vi "ForceAnnotationAuto.vi"(4 "EnReturnForce":bool, 5 "EnFullAngle":bool, 6 "SpectConfig":T4, 7 "FirstTouch":T3={"FirstPeakforce"=2.0, "F_LengthView"=20, "A_LengthView "=20} {"FirstPeakforce" format="%#_13g"}, 8 "ShowName":cluster{"ShowArrow":bool, "Alias":bool}, 9 "Test Name":string(combo)="WDW", 10 "Graph Up":refnum<vi>, 11 "Graph Down":refnum<vi>) -> (0 "MaxForceUp":T2, 1 "ResultUp":T1, 2 "ResultDown":T1, 3 "MaxForceDown":T2)   [LabVIEW 2017]
uses:
  <vilib>/Utility/miscctls.llb/LVAnnotationListTypeDef.ctl
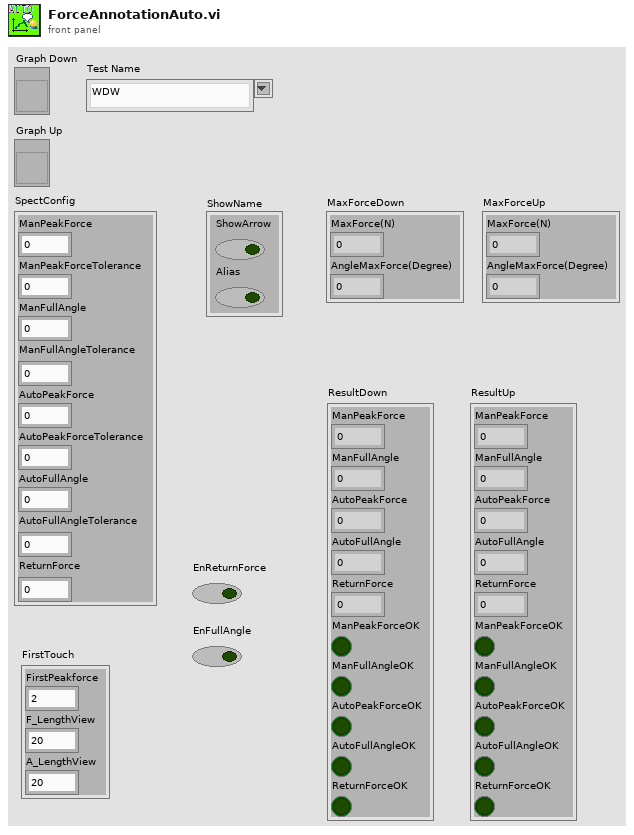
[diagram p1: front panel]
types:
  T1 = cluster{"ManPeakForce":dbl, "ManFullAngle":dbl, "AutoPeakForce":dbl, "AutoFullAngle":dbl, "ReturnForce":dbl, "ManPeakForceOK":bool, "ManFullAngleOK":bool, "AutoPeakForceOK":bool, "AutoFullAngleOK":bool, "ReturnForceOK":bool}
  T2 = cluster{"MaxForce(N)":dbl, "AngleMaxForce(Degree)":dbl}
  T3 = cluster{"FirstPeakforce":dbl, "F_LengthView":i32, "A_LengthView ":i32}
  T4 = cluster{"ManPeakForce":dbl, "ManPeakForceTolerance":dbl, "ManFullAngle":dbl, "ManFullAngleTolerance":dbl, "AutoPeakForce":dbl, "AutoPeakForceTolerance":dbl, "AutoFullAngle":dbl, "AutoFullAngleTolerance":dbl, "ReturnForce":dbl}
  T5 = cluster{"FirstForce":dbl, "LengthView":i32, "Name":string}
  T6 = typedef "LVAnnotationListTypeDef.ctl" = cluster{"Name":string, "Color":u32, "Style":u8, "Point Style":u8, "Name Visible":bool, "Allow Drag":bool, "Annotation Mode":u32, "Plot":i32, "Index":i32, "Position":cluster{"X":dbl, "Y":dbl}, "X Scale":u32, "Y Scale":u32, "Show Arrow":bool, "Lock Name":bool, "Plot Area":i32, "Label Offset":cluster{"X":dbl, "Y":dbl}}[]
  T7 = cluster{"Annotation List[0]":cluster{"Name":string, "Color":u32, "Style":u8, "Point Style":u8, "Name Visible":bool, "Allow Drag":bool, "Annotation Mode":u32, "Plot":i32, "Index":i32, "Position":cluster{"X":dbl, "Y":dbl}, "X Scale":u32, "Y Scale":u32, "Show Arrow":bool, "Lock Name":bool, "Plot Area":i32, "Label Offset":cluster{"X":dbl, "Y":dbl}}, "Annotation List[1]":cluster{"Name":string, "Color":u32, "Style":u8, "Point Style":u8, "Name Visible":bool, "Allow Drag":bool, "Annotation Mode":u32, "Plot":i32, "Index":i32, "Position":cluster{"X":dbl, "Y":dbl}, "X Scale":u32, "Y Scale":u32, "Show Arrow":bool, "Lock Name":bool, "Plot Area":i32, "Label Offset":cluster{"X":dbl, "Y":dbl}}, "Annotation List[2]":cluster{"Name":string, "Color":u32, "Style":u8, "Point Style":u8, "Name Visible":bool, "Allow Drag":bool, "Annotation Mode":u32, "Plot":i32, "Index":i32, "Position":cluster{"X":dbl, "Y":dbl}, "X Scale":u32, "Y Scale":u32, "Show Arrow":bool, "Lock Name":bool, "Plot Area":i32, "Label Offset":cluster{"X":dbl, "Y":dbl}}, "Annotation List[3]":cluster{"Name":string, "Color":u32, "Style":u8, "Point Style":u8, "Name Visible":bool, "Allow Drag":bool, "Annotation Mode":u32, "Plot":i32, "Index":i32, "Position":cluster{"X":dbl, "Y":dbl}, "X Scale":u32, "Y Scale":u32, "Show Arrow":bool, "Lock Name":bool, "Plot Area":i32, "Label Offset":cluster{"X":dbl, "Y":dbl}}, "Annotation List[4]":cluster{"Name":string, "Color":u32, "Style":u8, "Point Style":u8, "Name Visible":bool, "Allow Drag":bool, "Annotation Mode":u32, "Plot":i32, "Index":i32, "Position":cluster{"X":dbl, "Y":dbl}, "X Scale":u32, "Y Scale":u32, "Show Arrow":bool, "Lock Name":bool, "Plot Area":i32, "Label Offset":cluster{"X":dbl, "Y":dbl}}, "Annotation List[5]":cluster{"Name":string, "Color":u32, "Style":u8, "Point Style":u8, "Name Visible":bool, "Allow Drag":bool, "Annotation Mode":u32, "Plot":i32, "Index":i32, "Position":cluster{"X":dbl, "Y":dbl}, "X Scale":u32, "Y Scale":u32, "Show Arrow":bool, "Lock Name":bool, "Plot Area":i32, "Label Offset":cluster{"X":dbl, "Y":dbl}}, "Annotation List[6]":cluster{"Name":string, "Color":u32, "Style":u8, "Point Style":u8, "Name Visible":bool, "Allow Drag":bool, "Annotation Mode":u32, "Plot":i32, "Index":i32, "Position":cluster{"X":dbl, "Y":dbl}, "X Scale":u32, "Y Scale":u32, "Show Arrow":bool, "Lock Name":bool, "Plot Area":i32, "Label Offset":cluster{"X":dbl, "Y":dbl}}, "Annotation List[7]":cluster{"Name":string, "Color":u32, "Style":u8, "Point Style":u8, "Name Visible":bool, "Allow Drag":bool, "Annotation Mode":u32, "Plot":i32, "Index":i32, "Position":cluster{"X":dbl, "Y":dbl}, "X Scale":u32, "Y Scale":u32, "Show Arrow":bool, "Lock Name":bool, "Plot Area":i32, "Label Offset":cluster{"X":dbl, "Y":dbl}}, "Annotation List[8]":cluster{"Name":string, "Color":u32, "Style":u8, "Point Style":u8, "Name Visible":bool, "Allow Drag":bool, "Annotation Mode":u32, "Plot":i32, "Index":i32, "Position":cluster{"X":dbl, "Y":dbl}, "X Scale":u32, "Y Scale":u32, "Show Arrow":bool, "Lock Name":bool, "Plot Area":i32, "Label Offset":cluster{"X":dbl, "Y":dbl}}}
  T8 = cluster{"Name":string, "Color":u32, "Style":u8, "Point Style":u8, "Name Visible":bool, "Allow Drag":bool, "Annotation Mode":u32, "Plot":i32, "Index":i32, "Position":cluster{"X":dbl, "Y":dbl}, "X Scale":u32, "Y Scale":u32, "Show Arrow":bool, "Lock Name":bool, "Plot Area":i32, "Label Offset":cluster{"X":dbl, "Y":dbl}}[]
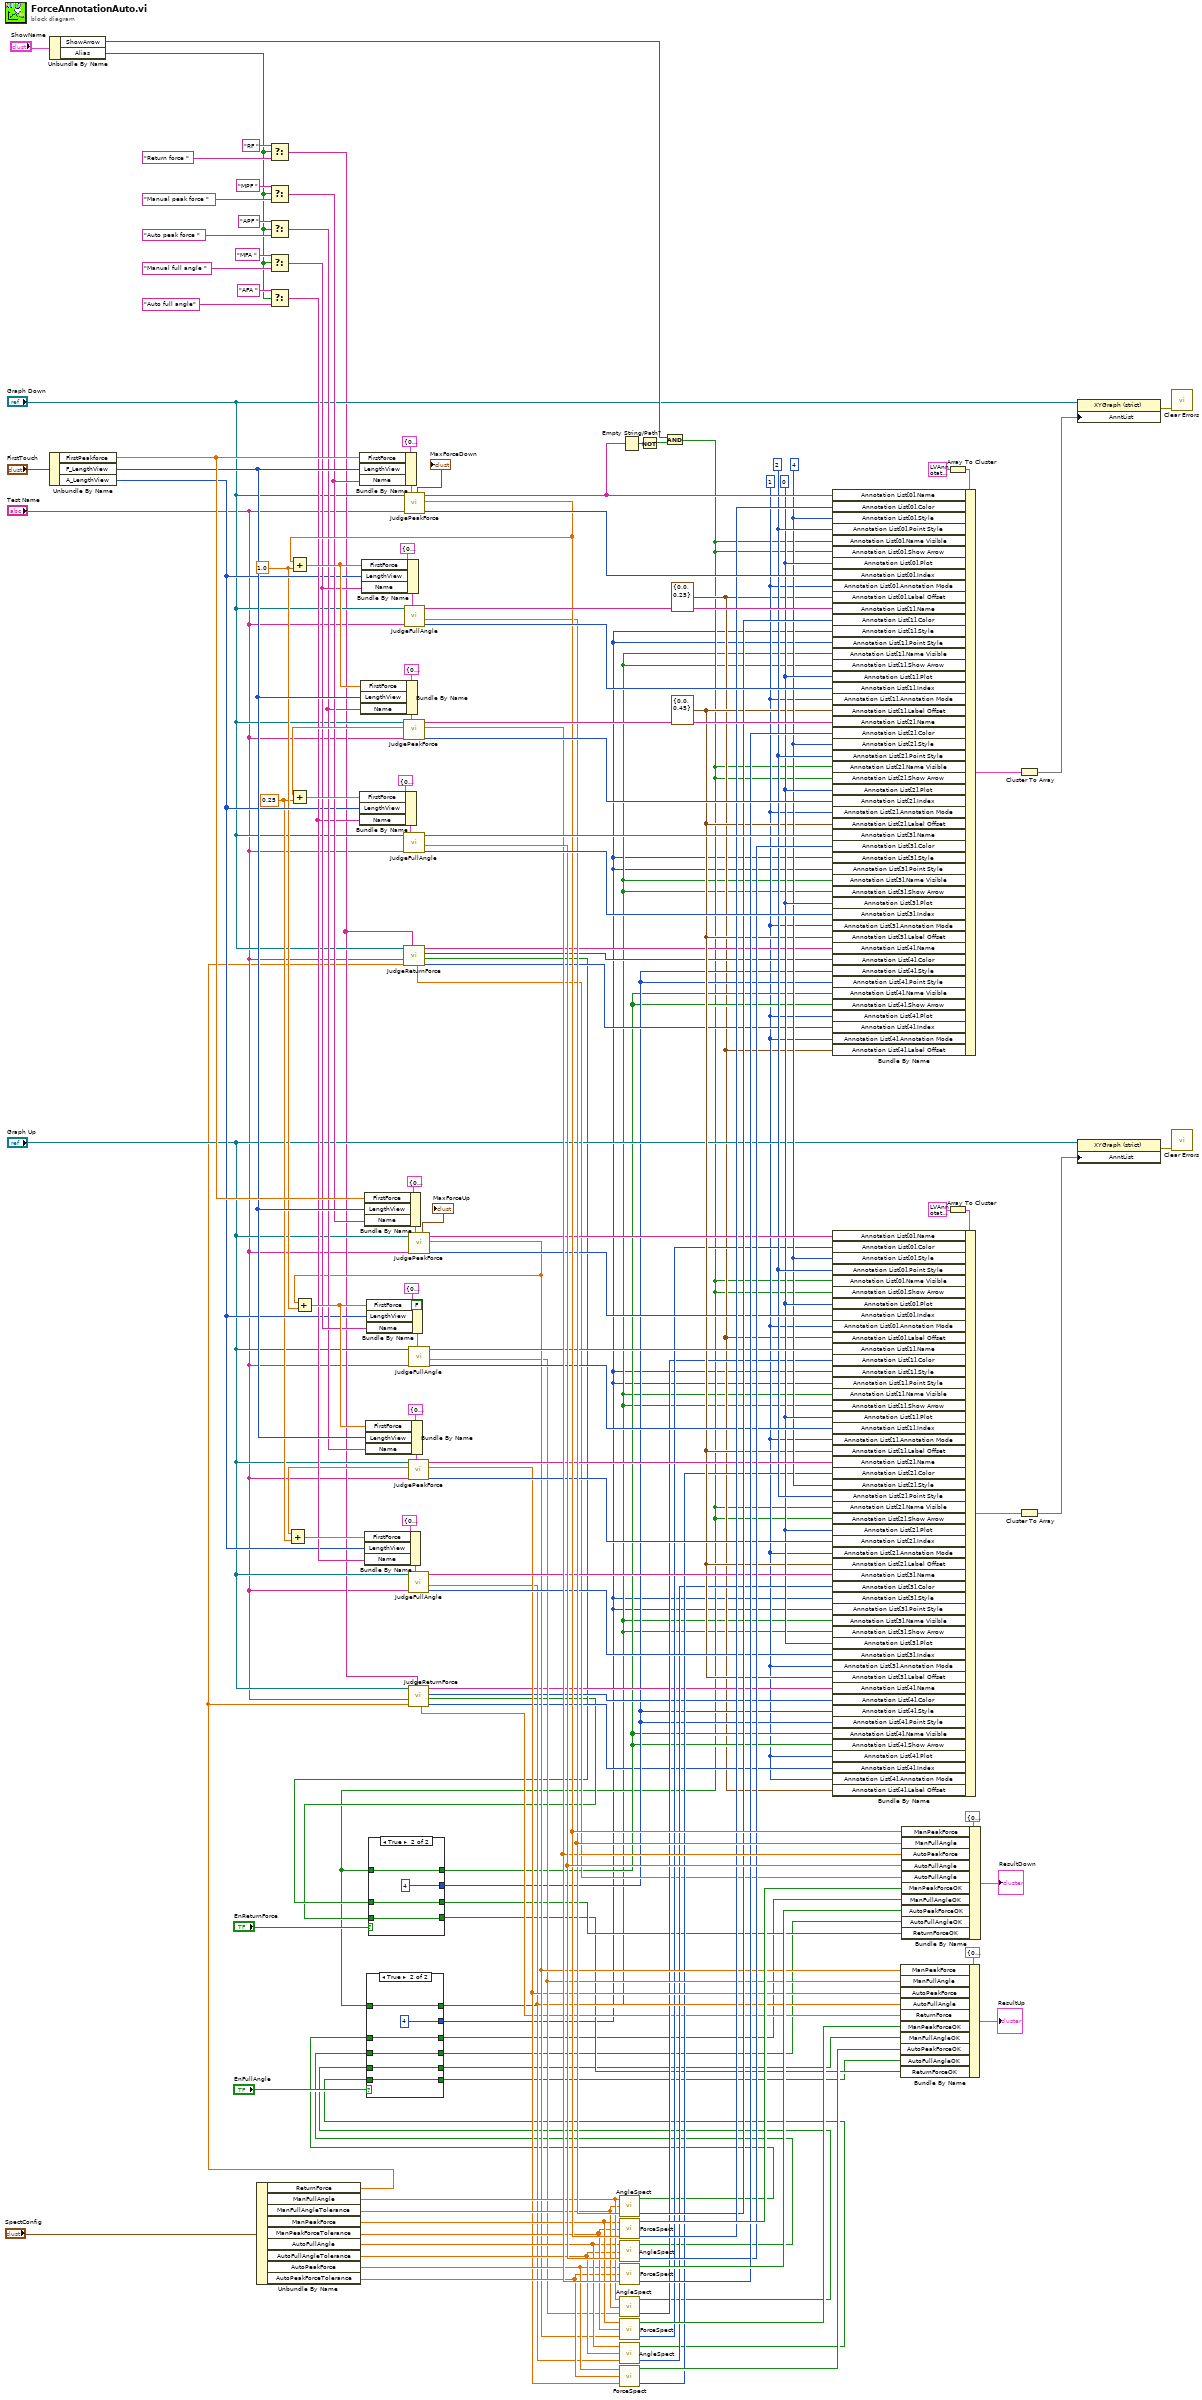
[diagram p0: block diagram]
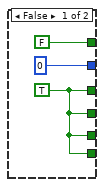
[diagram p2: hidden frame]
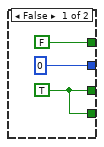
[diagram p3: hidden frame]
diagram:
  (unwired) FALSE ("Auto")
  w71 = 0 ("Annotation List[0].Plot")
  w69 = cluster{"X":dbl, "Y":dbl} {"X"=0.0, "Y"=0.45} ("Annotation List[0].Label Offset")
  w42 = 0.25 ("y")
  w43 = 1.0 ("y")
  w72 = u8 2 ("Annotation List[0].Point Style")
  w17 = cluster{"X":dbl, "Y":dbl} {"X"=0.0, "Y"=0.25} ("Annotation List[0].Label Offset")
  w18 = u32 1 ("Annotation List[0].Annotation Mode")
  w70 = u8 4 ("Annotation List[0].Style")
  n1 = Unbundle By Name("FirstTouch") -> ("FirstPeakforce"=w68:dbl, "F_LengthView"=w67:i32, "A_LengthView"=w62:i32)
  n2 = Unbundle By Name("ShowName") -> ("ShowArrow"=w127:bool, "Alias"=w38:bool)
  n3 = Unbundle By Name("SpectConfig") -> ("ReturnForce"=w25:dbl, "ManFullAngle"=w61:dbl, "ManFullAngleTolerance"=w60:dbl, "ManPeakForce"=w59:dbl, "ManPeakForceTolerance"=w58:dbl, "AutoFullAngle"=w57:dbl, "AutoFullAngleTolerance"=w56:dbl, "AutoPeakForce"=w55:dbl, "AutoPeakForceTolerance"=w54:dbl)
  n4 = Select(t="RF ", s=w38, f="Return force " ("Name")) -> (s? t:f=w27:string)
  n5 = Select(t="MPF ", s=w38, f="Manual peak force " ("Name")) -> (s? t:f=w66:string)
  n6 = Select(t="APF ", s=w38, f="Auto peak force " ("Name")) -> (s? t:f=w64:string)
  n7 = Select(t="MFA ", s=w38, f="Manual full angle " ("Name")) -> (s? t:f=w65:string)
  n8 = Select(t="AFA ", s=w38, f="Auto full angle" ("Name")) -> (s? t:f=w63:string)
  n9 = Bundle By Name(cluster=T5 {"FirstForce"=0.18, "LengthView"=30, "Name"="Peak Force"} ("Config"), "FirstForce"=w68, "LengthView"=w67, "Name"=w66) -> (w112:T5)
  n10 = Bundle By Name(cluster=T5 {"FirstForce"=0.18, "LengthView"=30, "Name"="Peak Force"} ("Config"), "FirstForce"=w68, "LengthView"=w67, "Name"=w66) -> (w88:T5)
  n11 = call "JudgeReturnForce.vi"("Name"=w27, "ReturnForce"=w25, "Test Name"="Test Name", "GraphDown"="Graph Down") -> ("IndexOut"=w29:i32, "Result"=w16:bool, "ColorResult"=w30:u32, "ReturnForceValue"=w31:string, "ReturnForce"=w32:dbl)  [unwired: 3 in]
  n12 = call "JudgePeakForce.vi"("Config"=w112, "Test Name"="Test Name", "XYGraph"="Graph Down") -> ("IndexOut"=w140:i32, "ForceOut"=w107:dbl, "Force Value"=w142:string, "MaxForce"=→"MaxForceDown":T2)  [unwired: 4 in, 1 out]
  n13 = Add(x=w107, y=w43) -> (x+y=w106:dbl)
  n14 = Bundle By Name(cluster=T5 {"FirstForce"=0.18, "LengthView"=30, "Name"="Peak Force"} ("Config"), "FirstForce"=w106, "LengthView"=w67, "Name"=w64) -> (w108:T5)
  n15 = Bundle By Name(cluster=T5 {"FirstForce"=0.18, "LengthView"=30, "Name"="Full Angle "} ("Config"), "FirstForce"=w106, "LengthView"=w62, "Name"=w65) -> (w110:T5)
  n16 = call "JudgePeakForce.vi"("Config"=w108, "Test Name"="Test Name", "XYGraph"="Graph Down") -> ("IndexOut"=w132:i32, "ForceOut"=w101:dbl, "Force Value"=w133:string)  [unwired: 4 in, 2 out]
  n17 = Add(x=w101, y=w42) -> (x+y=w103:dbl)
  n18 = Bundle By Name(cluster=T5 {"FirstForce"=0.18, "LengthView"=30, "Name"="Full Angle "} ("Config"), "FirstForce"=w103, "LengthView"=w62, "Name"=w63) -> (w104:T5)
  n19 = call "JudgeFullAngle.vi"("Config"=w104, "Test Name"="Test Name", "XYGraph"="Graph Down") -> ("IndexOut"=w130:i32, "AngleOut"=w117:dbl, "Force Value"=w131:string)  [unwired: 5 in, 1 out]
  n20 = call "JudgeFullAngle.vi"("Config"=w110, "Test Name"="Test Name", "XYGraph"="Graph Down") -> ("IndexOut"=w134:i32, "AngleOut"=w102:dbl, "Force Value"=w135:string)  [unwired: 5 in, 1 out]
  n21 = call "JudgeReturnForce.vi"("Name"=w27, "ReturnForce"=w25, "Test Name"="Test Name", "GraphDown"="Graph Up") -> ("IndexOut"=w19:i32, "Result"=w14:bool, "ColorResult"=w23:u32, "ReturnForceValue"=w24:string, "ReturnForce"=w22:dbl)  [unwired: 3 in]
  n22 = call "JudgePeakForce.vi"("Config"=w88, "Test Name"="Test Name", "XYGraph"="Graph Up") -> ("IndexOut"=w75:i32, "ForceOut"=w53:dbl, "Force Value"=w73:string, "MaxForce"=→"MaxForceUp":T2)  [unwired: 4 in, 1 out]
  n23 = Add(x=w53, y=w43) -> (x+y=w93:dbl)
  n24 = Bundle By Name(cluster=T5 {"FirstForce"=0.18, "LengthView"=30, "Name"="Peak Force"} ("Config"), "FirstForce"=w93, "LengthView"=w67, "Name"=w64) -> (w92:T5)
  n25 = Bundle By Name(cluster=T5 {"FirstForce"=0.18, "LengthView"=30, "Name"="Full Angle "} ("Config"), "FirstForce"=w93, "LengthView"=w62, "Name"=w65) -> (w90:T5)
  n26 = call "JudgePeakForce.vi"("Config"=w92, "Test Name"="Test Name", "XYGraph"="Graph Up") -> ("IndexOut"=w83:i32, "ForceOut"=w51:dbl, "Force Value"=w82:string)  [unwired: 4 in, 2 out]
  n27 = Add(x=w51, y=w42) -> (x+y=w96:dbl)
  n28 = Bundle By Name(cluster=T5 {"FirstForce"=0.18, "LengthView"=30, "Name"="Full Angle "} ("Config"), "FirstForce"=w96, "LengthView"=w62, "Name"=w63) -> (w95:T5)
  n29 = call "JudgeFullAngle.vi"("Config"=w95, "Test Name"="Test Name", "XYGraph"="Graph Up") -> ("IndexOut"=w85:i32, "AngleOut"=w50:dbl, "Force Value"=w84:string)  [unwired: 5 in, 1 out]
  n30 = call "JudgeFullAngle.vi"("Config"=w90, "Test Name"="Test Name", "XYGraph"="Graph Up") -> ("IndexOut"=w81:i32, "AngleOut"=w52:dbl, "Force Value"=w80:string)  [unwired: 5 in, 1 out]
  n31 = call "AngleSpect.vi"("Angle In"=w102, "Angle Tolerance"=w60, "Angle  Spect"=w61) -> ("Angle Color"=w99:u32, "Angle OK"=w8:bool)  [unwired: 1 in]
  n32 = call "ForceSpect.vi"("Force Input"=w107, "Force Tolerance"=w58, "Force  Spect"=w59) -> ("Force Color"=w100:u32, "Force OK"=w116:bool)  [unwired: 1 in]
  n33 = call "AngleSpect.vi"("Angle In"=w117, "Angle Tolerance"=w56, "Angle  Spect"=w57) -> ("Angle Color"=w97:u32, "Angle OK"=w6:bool)  [unwired: 1 in]
  n34 = call "ForceSpect.vi"("Force Input"=w101, "Force Tolerance"=w54, "Force  Spect"=w55) -> ("Force Color"=w98:u32, "Force OK"=w115:bool)  [unwired: 1 in]
  n35 = call "AngleSpect.vi"("Angle In"=w52, "Angle Tolerance"=w60, "Angle  Spect"=w61) -> ("Angle Color"=w46:u32, "Angle OK"=w4:bool)  [unwired: 1 in]
  n36 = call "ForceSpect.vi"("Force Input"=w53, "Force Tolerance"=w58, "Force  Spect"=w59) -> ("Force Color"=w47:u32, "Force OK"=w49:bool)  [unwired: 1 in]
  n37 = call "AngleSpect.vi"("Angle In"=w50, "Angle Tolerance"=w56, "Angle  Spect"=w57) -> ("Angle Color"=w44:u32, "Angle OK"=w2:bool)  [unwired: 1 in]
  n38 = call "ForceSpect.vi"("Force Input"=w51, "Force Tolerance"=w54, "Force  Spect"=w55) -> ("Force Color"=w45:u32, "Force OK"=w48:bool)  [unwired: 1 in]
  n39 = Empty String/Path?(string/path=w142) -> (empty?=w143:bool)
  n40 = Not(x=w143) -> (.not. x?=w144:bool)
  n41 = And(x=w127, y=w144) -> (x .and. y?=w11:bool)
  n42 = case shown="True" "EnFullAngle" {
    tunnel: [0 4] -> w9
    tunnel: [FALSE w152] -> w10
    tunnel: w11 -> [_ w152]
    tunnel: [w145 w151] -> w7
    tunnel: [w145 w150] -> w5
    tunnel: w8 -> [_ w151]
    tunnel: w6 -> [_ w150]
    tunnel: [w145 w149] -> w3
    tunnel: [w145 w148] -> w1
    tunnel: w4 -> [_ w149]
    tunnel: w2 -> [_ w148]
    frame False {
      w145 = TRUE ("Result")
    }
    frame True {
    }
  }
  n43 = case shown="True" "EnReturnForce" {
    tunnel: [0 4] -> w21
    tunnel: [FALSE w159] -> w20
    tunnel: w11 -> [_ w159]
    tunnel: w16 -> [_ w158]
    tunnel: [w154 w158] -> w15
    tunnel: w14 -> [_ w157]
    tunnel: [w154 w157] -> w13
    frame False {
      w154 = TRUE ("Result")
    }
    frame True {
    }
  }
  n44 = Bundle By Name(cluster=T1 {"ManPeakForce"=0.0, "ManFullAngle"=0.0, "AutoPeakForce"=0.0, "AutoFullAngle"=0.0, "ReturnForce"=0.0, "ManPeakForceOK"=FALSE, "ManFullAngleOK"=FALSE, "AutoPeakForceOK"=FALSE, "AutoFullAngleOK"=FALSE, "ReturnForceOK"=FALSE} ("ResultDown"), "ManPeakForce"=w53, "ManFullAngle"=w52, "AutoPeakForce"=w51, "AutoFullAngle"=w50, "ReturnForce"=w22, "ManPeakForceOK"=w49, "ManFullAngleOK"=w3, "AutoPeakForceOK"=w48, "AutoFullAngleOK"=w1, "ReturnForceOK"=w13) -> (→"ResultUp":T1)
  n45 = Bundle By Name(cluster=T1 {"ManPeakForce"=0.0, "ManFullAngle"=0.0, "AutoPeakForce"=0.0, "AutoFullAngle"=0.0, "ReturnForce"=0.0, "ManPeakForceOK"=FALSE, "ManFullAngleOK"=FALSE, "AutoPeakForceOK"=FALSE, "AutoFullAngleOK"=FALSE, "ReturnForceOK"=FALSE} ("ResultDown"), "ManPeakForce"=w107, "ManFullAngle"=w102, "AutoPeakForce"=w101, "AutoFullAngle"=w117, "AutoFullAngle"=w32, "ManPeakForceOK"=w116, "ManFullAngleOK"=w7, "AutoPeakForceOK"=w115, "AutoFullAngleOK"=w5, "ReturnForceOK"=w15) -> (→"ResultDown":T1)
  n46 = Array To Cluster(array=T6 [{"Name"="", "Color"=0, "Style"=0, "Point Style"=0, "Name Visible"=FALSE, "Allow Drag"=FALSE, "Annotation Mode"=0, "Plot"=0, "Index"=0, "Position"={"X"=0.0, "Y"=0.0}, "X Scale"=0, "Y Scale"=0, "Show Arrow"=FALSE, "Lock Name"=FALSE, "Plot Area"=0, "Label Offset"={"X"=0.0, "Y"=0.0}}] ("Annotation List")) -> (cluster=w137:T7)
  n47 = Bundle By Name(cluster=w137, "Annotation List[0].Name"=w142, "Annotation List[0].Color"=w100, "Annotation List[0].Style"=w70, "Annotation List[0].Point Style"=w72, "Annotation List[0].Name Visible"=w11, "Annotation List[0].Show Arrow"=w11, "Annotation List[0].Plot"=w71, "Annotation List[0].Index"=w140, "Annotation List[0].Annotation Mode"=w18, "Annotation List[0].Label Offset"=w17, "Annotation List[1].Name"=w135, "Annotation List[1].Color"=w99, "Annotation List[1].Style"=w9, "Annotation List[1].Point Style"=w9, "Annotation List[1].Name Visible"=w10, "Annotation List[1].Show Arrow"=w10, "Annotation List[1].Plot"=w71, "Annotation List[1].Index"=w134, "Annotation List[1].Annotation Mode"=w18, "Annotation List[1].Label Offset"=w69, "Annotation List[2].Name"=w133, "Annotation List[2].Color"=w98, "Annotation List[2].Style"=w70, "Annotation List[2].Point Style"=w72, "Annotation List[2].Name Visible"=w11, "Annotation List[2].Show Arrow"=w11, "Annotation List[2].Plot"=w71, "Annotation List[2].Index"=w132, "Annotation List[2].Annotation Mode"=w18, "Annotation List[2].Label Offset"=w69, "Annotation List[3].Name"=w131, "Annotation List[3].Color"=w97, "Annotation List[3].Style"=w9, "Annotation List[3].Point Style"=w9, "Annotation List[3].Name Visible"=w10, "Annotation List[3].Show Arrow"=w10, "Annotation List[3].Plot"=w71, "Annotation List[3].Index"=w130, "Annotation List[3].Annotation Mode"=w18, "Annotation List[3].Label Offset"=w69, "Annotation List[4].Name"=w31, "Annotation List[4].Color"=w30, "Annotation List[4].Style"=w21, "Annotation List[4].Point Style"=w21, "Annotation List[4].Name Visible"=w20, "Annotation List[4].Show Arrow"=w20, "Annotation List[4].Plot"=w18, "Annotation List[4].Index"=w29, "Annotation List[4].Annotation Mode"=w18, "Annotation List[4].Label Offset"=w17) -> (w138:T7)
  n48 = Array To Cluster(array=T6 [{"Name"="", "Color"=0, "Style"=0, "Point Style"=0, "Name Visible"=FALSE, "Allow Drag"=FALSE, "Annotation Mode"=0, "Plot"=0, "Index"=0, "Position"={"X"=0.0, "Y"=0.0}, "X Scale"=0, "Y Scale"=0, "Show Arrow"=FALSE, "Lock Name"=FALSE, "Plot Area"=0, "Label Offset"={"X"=0.0, "Y"=0.0}}] ("Annotation List")) -> (cluster=w78:T7)
  n49 = Bundle By Name(cluster=w78, "Annotation List[0].Name"=w73, "Annotation List[0].Color"=w47, "Annotation List[0].Style"=w70, "Annotation List[0].Point Style"=w72, "Annotation List[0].Name Visible"=w11, "Annotation List[0].Show Arrow"=w11, "Annotation List[0].Plot"=w71, "Annotation List[0].Index"=w75, "Annotation List[0].Annotation Mode"=w18, "Annotation List[0].Label Offset"=w17, "Annotation List[1].Name"=w80, "Annotation List[1].Color"=w46, "Annotation List[1].Style"=w9, "Annotation List[1].Point Style"=w9, "Annotation List[1].Name Visible"=w10, "Annotation List[1].Show Arrow"=w10, "Annotation List[1].Plot"=w71, "Annotation List[1].Index"=w81, "Annotation List[1].Annotation Mode"=w18, "Annotation List[1].Label Offset"=w69, "Annotation List[2].Name"=w82, "Annotation List[2].Color"=w45, "Annotation List[2].Style"=w70, "Annotation List[2].Point Style"=w72, "Annotation List[2].Name Visible"=w11, "Annotation List[2].Show Arrow"=w11, "Annotation List[2].Plot"=w71, "Annotation List[2].Index"=w83, "Annotation List[2].Annotation Mode"=w18, "Annotation List[2].Label Offset"=w69, "Annotation List[3].Name"=w84, "Annotation List[3].Color"=w44, "Annotation List[3].Style"=w9, "Annotation List[3].Point Style"=w9, "Annotation List[3].Name Visible"=w10, "Annotation List[3].Show Arrow"=w10, "Annotation List[3].Plot"=w71, "Annotation List[3].Index"=w85, "Annotation List[3].Annotation Mode"=w18, "Annotation List[3].Label Offset"=w69, "Annotation List[4].Name"=w24, "Annotation List[4].Color"=w23, "Annotation List[4].Style"=w21, "Annotation List[4].Point Style"=w21, "Annotation List[4].Name Visible"=w20, "Annotation List[4].Show Arrow"=w20, "Annotation List[4].Plot"=w18, "Annotation List[4].Index"=w19, "Annotation List[4].Annotation Mode"=w18, "Annotation List[4].Label Offset"=w17) -> (w77:T7)
  n50 = Cluster To Array(cluster=w138) -> (array=w139:T8)
  n51 = Cluster To Array(cluster=w77) -> (array=w76:T8)
  n52 = property on="Property Node" class="XYGraph (strict)"(reference="Graph Down", "AnntList"=w139) -> (error out=w141:errorcluster)  [unwired: 1 in, 1 out]
  n53 = property on="Property Node" class="XYGraph (strict)"(reference="Graph Up", "AnntList"=w76) -> (error out=w74:errorcluster)  [unwired: 1 in, 1 out]
  n54 = call <vilib>:"Clear Errors.vi"("error in (no error)"=w141) -> ()  [unwired: 5 in, 2 out]
  n55 = call <vilib>:"Clear Errors.vi"("error in (no error)"=w74) -> ()  [unwired: 5 in, 2 out]
